vi "Perf Meter.vi"() -> ()   [LabVIEW 2025]
doc: "Author: Scott Hannahs <sth@magnet.fsu.edu>\n\nThis software is licensed for use under the “MIT License\"\nCopyright (c) 2025 Scott Hannahs, sth@sth@magnet.sthnet.net\n\nPermission is hereby granted, free of charge, to any person obtaining a copy of this software and associated documentation files (the \"Software\"), to deal in the Software without restriction, including without limitation the rights to use, copy, modify, merge, publish, distribute, sublicense, and/or sell copies of the Software, and to permit persons to whom the Software is furnished to do so, subject to the following conditions: The above copyright notice and this permission notice shall be included in all copies or substantial portions of the Software.\n\nTHE SOFTWARE IS PROVIDED \"AS IS\", WITHOUT WARRANTY OF ANY KIND, EXPRESS OR IMPLIED, INCLUDING BUT NOT LIMITED TO THE WARRANTIES OF MERCHANTABILITY, FITNESS FOR A PARTICULAR PURPOSE AND NONINFRINGEMENT. IN NO EVENT SHALL THE AUTHORS OR COPYRIGHT HOLDERS BE LIABLE FOR ANY CLAIM, DAMAGES OR OTHER LIABILITY, WHETHER IN AN ACTION OF CONTRACT, TORT OR OTHERWISE, ARISING FROM, OUT OF OR IN CONNECTION WITH THE SOFTWARE OR THE USE OR OTHER DEALINGS IN THE SOFTWARE."
panel:
  out "Cycles / Sec":dbl(knob) scale=10000.0..1000000000.0
  in  "stop":bool
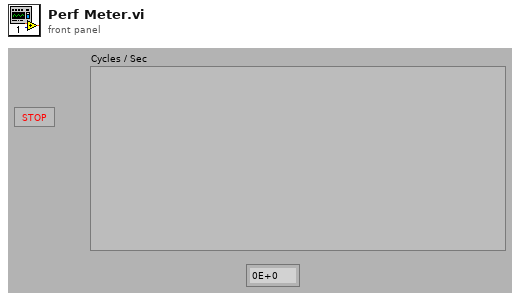
[diagram p1: front panel]
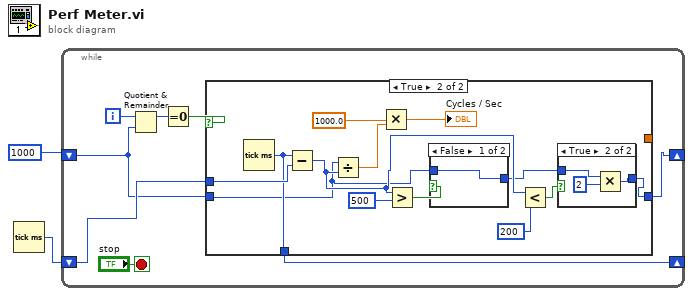
[diagram p0: block diagram]
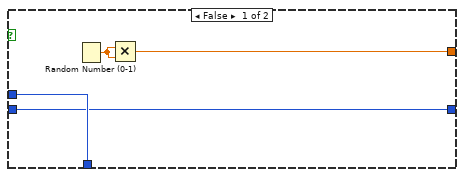
[diagram p2: hidden frame]
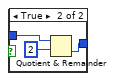
[diagram p4: hidden frame]
diagram:
  n1 = Tick Count (ms)() -> (millisecond timer value=w2:u32)
  n2 = while {
    shift-right: [w5] -> _
    shift-left: w2 -> [w6]
    shift-right: [w3] -> _
    shift-left: u32 1000 -> [w4]
    i -> [w9]
    stop <- "stop" stop-if-true
    n3 = Quotient & Remainder(x=w9, y=w4) -> (x-y*floor(x/y)=w8:u32)  [unwired: 1 out]
    n4 = Equal To 0?(x=w8) -> (x = 0?=w7:bool)
    n5 = case shown="True" w7 {
      tunnel: w6 -> [w14 w27]
      tunnel: [w14 w26] -> w5
      tunnel: w4 -> [w11 w17]
      tunnel: [w12 _] -> _
      tunnel: [w11 w18] -> w3
      frame False {
        n6 = Random Number (0-1)() -> (number: 0 to 1=w13:dbl)
        n7 = Multiply(x=w13, y=w13) -> (x*y=w12:dbl)
      }
      frame True {
        n8 = Tick Count (ms)() -> (millisecond timer value=w26:u32)
        n9 = Subtract(x=w26, y=w27) -> (x-y=w22:u32)
        n10 = Divide(x=w17, y=w22) -> (x/y=w25:dbl)
        n11 = Multiply(x=1000.0, y=w25) -> (x*y=→"Cycles / Sec":dbl)
        n12 = Greater?(x=w22, y=u32 500) -> (0:w23:bool)
        n13 = case shown="False" w23 {
          tunnel: w17 -> [w32 w35]
          tunnel: [w32 w33] -> w19
          frame False {
          }
          frame True {
            n14 = Quotient & Remainder(x=w35, y=u32 2) -> (floor(x/y)=w33:u32)  [unwired: 1 out]
          }
        }
        n15 = Less?(x=w22, y=u32 200) -> (x < y?=w20:bool)
        n16 = case shown="True" w20 {
          tunnel: w19 -> [w28 w31]
          tunnel: [w28 w29] -> w18
          frame False {
          }
          frame True {
            n17 = Multiply(x=w31, y=u32 2) -> (x*y=w29:u32)
          }
        }
      }
    }
  }
